vi "Flatten FIFO Flags.vi"(11 "Flags":T1) -> (3 "FIFO Flags":u64)   [LabVIEW 2021, in "ChannelCommon.lvlib"]
uses:
  ChannelCommon.lvlib
  typedef/FIFO Flags.ctl
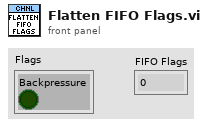
[diagram p1: front panel]
types:
  T1 = typedef "ChannelCommon.lvlib/FIFO Flags.ctl" = cluster{"Backpressure":bool}
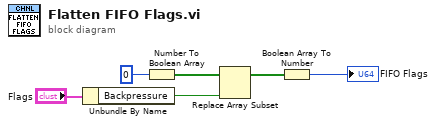
[diagram p0: block diagram]
diagram:
  n1 = Unbundle By Name("Flags") -> ("Backpressure"=w3:bool)
  n2 = Number To Boolean Array(number=u64 0) -> (Boolean array=w4:bool[])
  n3 = Replace Array Subset(array=w4, new element=w3) -> (w2:bool[])  [unwired: 1 in]
  n4 = Boolean Array To Number(Boolean array=w2) -> (number=→"FIFO Flags":u64)
